vi "YKMW100 Computation Control.vi"(0 "VISA session":refnum<visa-resource-name>="MW100", 5 "Mode":T1(ring), 11 "error in (no error)":errorcluster, 12 "Debug":bool) -> (4 "dup VISA session":refnum<visa-resource-name>="MW100", 15 "error out":errorcluster)   [LabVIEW 2023]
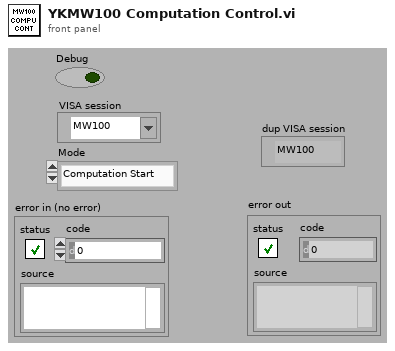
[diagram p1: front panel]
types:
  T1 = enum16{"Computation Start", "Computation stop", "Reset Computation", "Clear Computation"}
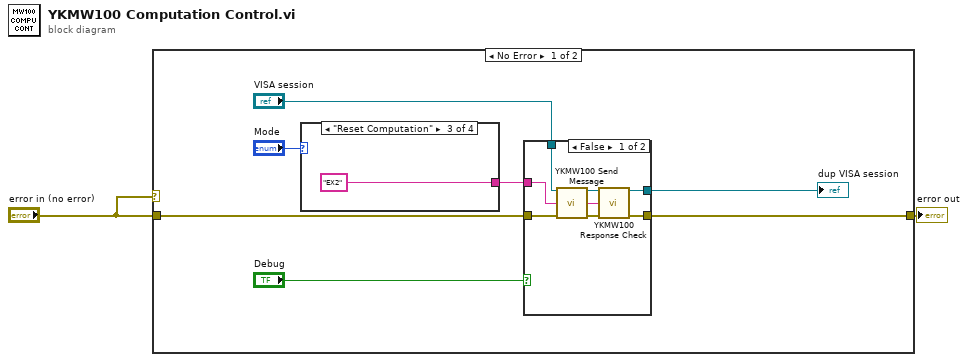
[diagram p0: block diagram]
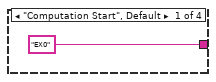
[diagram p3: hidden frame]
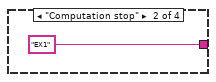
[diagram p4: hidden frame]
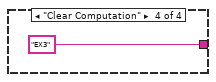
[diagram p5: hidden frame]
diagram:
  n1 = case shown="No Error" "error in (no error)" {
    tunnel: "error in (no error)" -> [w8 w24]
    tunnel: [w4 w24] -> w2
    frame No Error {
      n2 = case shown="\"Reset Computation\"" "Mode" {
        tunnel: ["EX0" ("Send Message (\"\")") "EX1" ("Send Message (\"\")") "EX2" ("Send Message (\"\")") "EX3" ("Send Message (\"\")")] -> w7
        frame "Computation Start", Default {
        }
        frame "Computation stop" {
        }
        frame "Reset Computation" {
        }
        frame "Clear Computation" {
        }
      }
      n3 = case shown="False" "Debug" {
        tunnel: w8 -> [w17 w18]
        tunnel: w7 -> [w16 _]
        tunnel: "VISA session" -> [w15 w19]
        tunnel: [w14 w19] -> w5
        tunnel: [w13 w18] -> w4
        frame False {
          n4 = call "YKMW100 Send Message.vi"("VISA session"=w15, "Send Message (\"\")"=w16, "error in (no error)"=w17) -> ("dup VISA session"=w10:refnum<visa-resource-name>, "Read Buffer"=w11:string, "error out"=w12:errorcluster)  [unwired: 10 in]
          n5 = call "YKMW100 Response Check.vi"("VISA session"=w10, "Message In (\"\")"=w11, "error in (no error)"=w12) -> ("dup VISA session"=w14:refnum<visa-resource-name>, "error out"=w13:errorcluster)  [unwired: 8 in, 3 out]
        }
        frame True {
        }
      }
      "dup VISA session" <- w5
    }
    frame Error {
    }
  }
  "error out" <- w2
